vi "DAQmx.44xx.Get Terminal Name with Device Prefix.vi"(8 "error in (no error)":errorcluster, 10 "Local Terminal Name":string, 11 "task":refnum<k21> caption="task/channels in") -> (0 "error out":errorcluster, 2 "Terminal Name with Device Prefix":tag, 3 "task out":refnum<k21>)   [LabVIEW 2019, in "DAQmx.lvclass"]
doc: "This example takes in a DAQmx Task and a terminal and converts this to a terminal which includes the device prefix specified in the DAQmx Physical Channel Control.\n\nFor example: \nDAQmx Task/channels in=Dev1/ai1:2\nTerminal=ai/StartTrigger\nDevice+Terminal=/Dev1/ai/StartTrigger"
uses:
  DAQmx.lvclass
  <resource>/objmgr/daqmx.rc
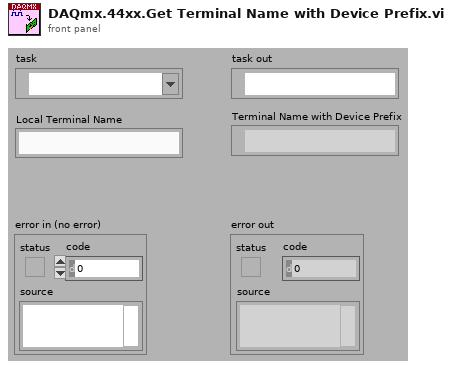
[diagram p1: front panel]
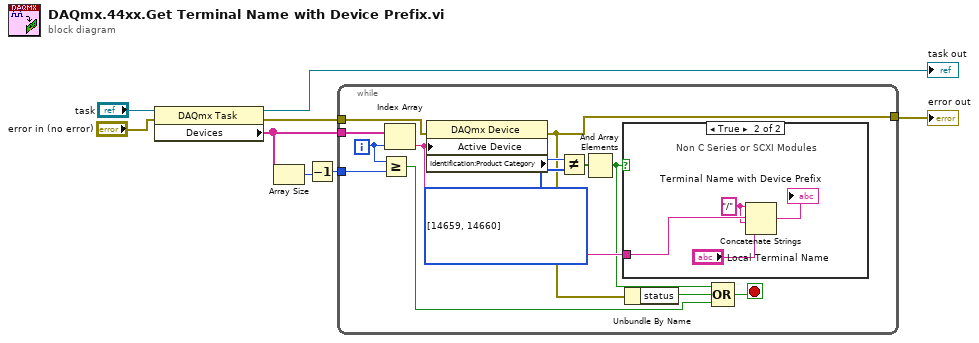
[diagram p0: block diagram]
diagram:
  n1 = property class="DAQmx Task"(reference="task", error in="error in (no error)") -> (reference out=→"task out":refnum<k21>, error out=w2:errorcluster, "Devices"=w3:tag[])
  n2 = Array Size(array=w3) -> (size(s)=w7:i32)
  n3 = Decrement(x=w7) -> (x-1=w6:i32)
  n4 = while {
    tunnel: w3 -> [w21]
    tunnel: w2 -> [w16]
    tunnel: [w15] -> w8
    tunnel: w6 -> [w13]
    i -> [w14]
    stop <- w9 stop-if-true
    w19 = i32[] [14659, 14660] items=["M Series DAQ"=14643, "E Series DAQ"=14642, "S Series DAQ"=14644, "B Series DAQ"=14662, "SC Series DAQ"=14645, "USB DAQ"=14646, "AO Series"=14647, "Digital I/O"=14648, "TIO Series"=14661, "Dynamic Signal Acquisition"=14649, "Switches"=14650, "C Series Chassis"=14658, "C Series Module"=14659, "SCXI Module"=14660, "Unknown"=12588]
    n5 = Greater Or Equal?(x=w14, y=w13) -> (x >= y?=w10:bool)
    n6 = Index Array(array=w21, index=w14) -> (element=w17:tag)
    n7 = property class="DAQmx Device"(error in=w16, "Active Device"=w17) -> (error out=w15:errorcluster, "Identification:Product Category"=w20:i32)  [unwired: 1 in, 1 out]
    n8 = Not Equal?(x=w20, y=w19) -> (x != y?=w18:bool[])
    n9 = And Array Elements(Boolean array=w18) -> (logical AND=w12:bool)
    n10 = case shown="True" w12 {
      tunnel: w17 -> [_ w25]
      frame False {
        # "Module Case do nothing"
      }
      frame True {
        w24 = "/" ("string")
        # "Non C Series or SCXI Modules"
        n11 = Concatenate Strings(w24, w25, w24, "Local Terminal Name") -> (→"Terminal Name with Device Prefix":string)
      }
    }
    n12 = Unbundle By Name(w15) -> ("status"=w11:bool)
    n13 = Compound Arithmetic op=OR(w12, w11, w10) -> (w9:bool)
  }
  "error out" <- w8
